vi "RRR_Joystick_Control_2025.vi"() -> ()   [LabVIEW 2020]
uses:
  <vilib>/MakerHub/LINX/Public/Peripherals/Analog/Analog Read N Chans.vi
  <vilib>/MakerHub/LINX/Public/Peripherals/Digital/Digital Read N Chans.vi
  <vilib>/MakerHub/LINX/Private/Local IO/LinxAnalogRead.vi
  <vilib>/MakerHub/LINX/Public/Utilities/Check Channel.vi
  <vilib>/MakerHub/LINX/Private/Local IO/LinxDigitalRead.vi
  <vilib>/MakerHub/LINX/Public/Utilities/Open Serial.vi
  <vilib>/MakerHub/LINX/Private/Utilties/Generate Error.vi
  <vilib>/MakerHub/LINX/LMH-LINX.lvlib
panel:
  out "Claw Angale":ext(slide) scale=0.0..1.0
  in  "Digital Channels":u8[](array[numeric])=[6, 7]
  in  "Analog Channels":u8[](array[numeric])=[0, 1, 2, 3]
  in  "Stop Button 2":bool
  out "Loop Rate (Hz) 2":u32=4294967295
  out "Voltages":dbl[](array[numeric])
  out "Values":bool[](array[boolean])
  out "Joint1_Theta":dbl=-2.0
  out "Joint2_Theta":dbl=-2.0
  out "Joint3_Theta":dbl=-2.0
  out "Claw_Theta":dbl=-2.0
  in  "Serial Port":refnum<visa-resource-name>="COM10"
  in  "Base position  Y":dbl
  in  "Base position X":dbl
  in  "Scale Factor":dbl(slide)=0.7 scale=0.5..1.0
  out "RRR - Forward Kinematics Visual":picture
  in  "Add details":bool=TRUE
  in  "Light Direction":dbl(knob)=5.611498737356196 scale format="%#.1f"
  in  "Colors":T1={"Joint 1"=16750848, "Arm 1"=16764006, "Joint 2"=26316, "Arm B"=6723993, "Joint 4"=16724787, "Claw"=16776960, "Joint 3"=26316, "Arm C"=6723993}
  out "TCP_Y":dbl=-5.928238312801877
  out "Joint2_Y":dbl=-3.8376690474488075
  out "Joint1_Y":dbl=-1.7449748351250485
  out "TCP_X":dbl=99.78690076611498
  out "Joint2_X":dbl=79.89646285874952
  out "Joint1_X":dbl=49.969541350954785
  in  "Arm 3":dbl=20.0
  out "RRR - Forward Kinematics":cluster{dbl[], dbl[]}(graph)={[0.0, 49.969541350954785, 79.89646285874952, 99.78690076611498], [39.0, -1.7449748351250485, -3.8376690474488075, -5.928238312801877]}
  in  "Arm 2":dbl=30.0
  in  "Arm 1":dbl=50.0
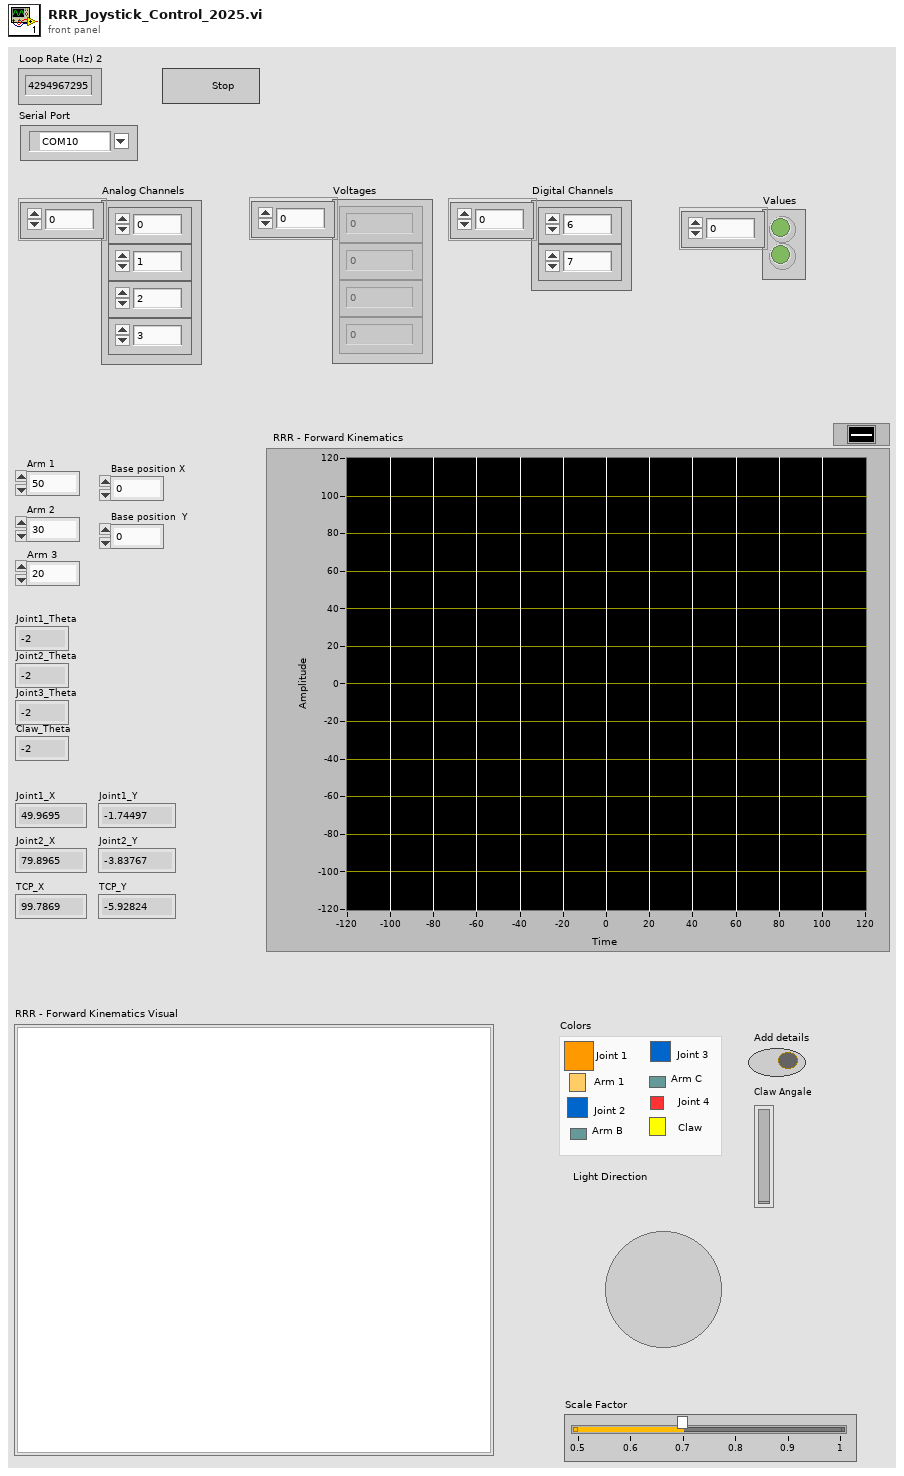
[diagram p1: front panel]
types:
  T1 = cluster{"Joint 1":u32, "Arm 1":u32, "Joint 2":u32, "Arm B":u32, "Joint 4":u32, "Claw":u32, "Joint 3":u32, "Arm C":u32}
  T2 = typedef "LMH-LINX.lvlib/LINX Ref.ctl" = cluster{"IO":T3, "Interface":T4, "LINX Device Config":T5}
  T3 = typedef "LMH-LINX.lvlib/Platform.ctl" = enum16{"Remote", "Local"}
  T4 = typedef "LMH-LINX.lvlib/Interface.ctl" = enum16{"Serial", "TCP"}
  T5 = typedef "LMH-LINX.lvlib/Device.lvlib/LINX Device Config.ctl" = cluster{"Interface":T4, "COM Port":refnum<visa-resource-name>, "TCP Configuration":T6, "Device Family":u8, "Device ID":u8, "Device Name":string, "TCP Ref":refnum<k5>, "Channels":T7}
  T6 = typedef "LMH-LINX.lvlib/Device.lvlib/TCP Config.ctl" = cluster{"IP Address":string, "Port":u16}
  T7 = typedef "LMH-LINX.lvlib/Channels.ctl" = cluster{"DI":u8[], "DO":u8[], "AI":u8[], "AO":u8[], "PWM":u8[], "QE":u8[], "UART":u8[], "I2C 2":u8[], "SPI":u8[], "CAN":u8[], "Servo":u8[], "AI Ref (V)":dbl, "AI Resolution (Bits)":u8, "AO Ref (V)":dbl, "AO Resolution (Bits)":u8}
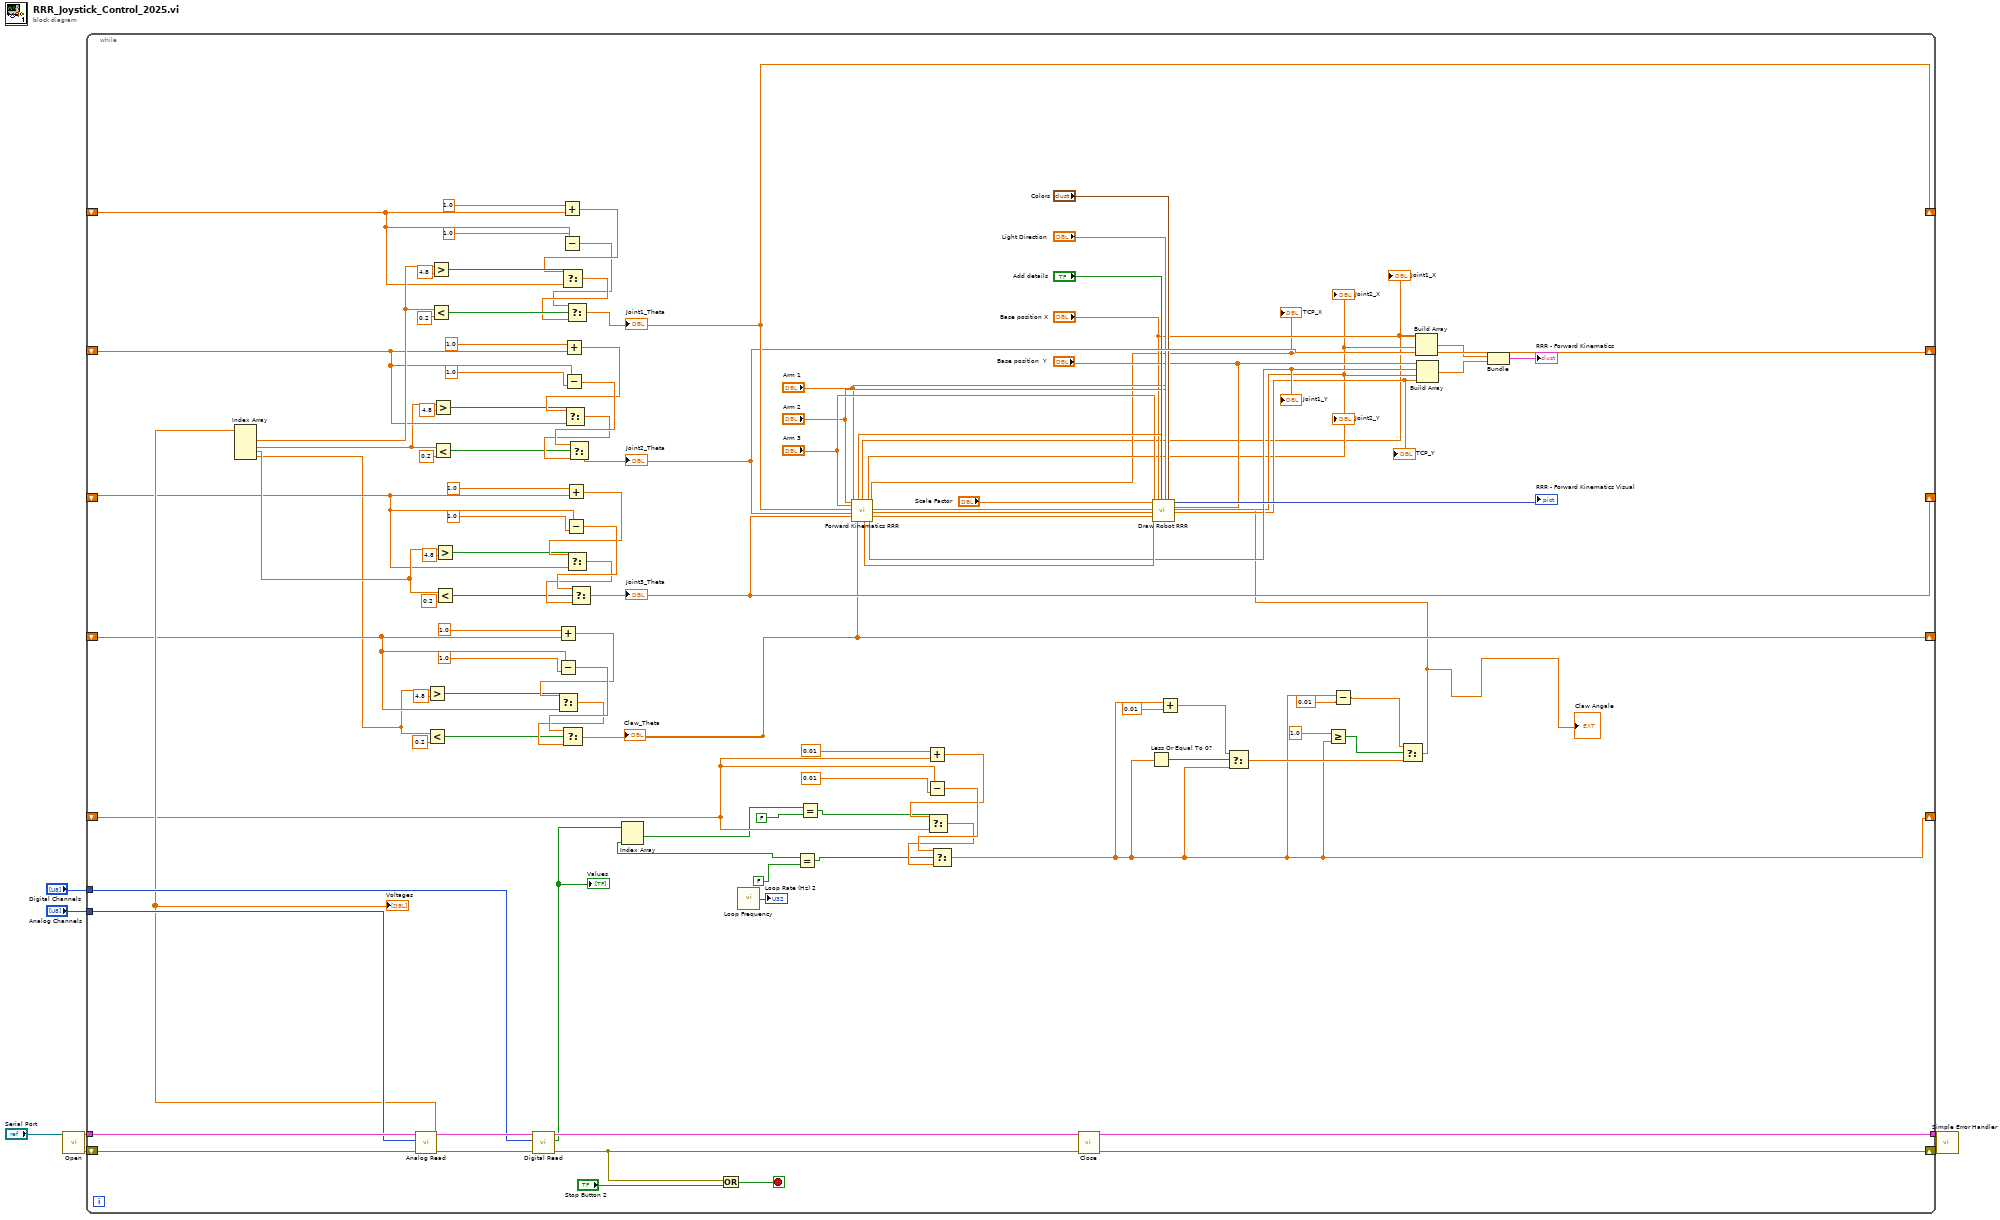
[diagram p0: block diagram]
diagram:
  n1 = call-poly <vilib>:"Open.vi"("Serial Port"="Serial Port") -> ("Error Out"=w7:errorcluster, "LINX Resource"=w8:T2)  [unwired: 8 in, 1 out]
  n2 = while {
    tunnel: w8 -> [w111]
    tunnel: [w108] -> w6
    shift-right: [w107] -> w5
    shift-left: w7 -> [w105]
    tunnel: "Analog Channels" -> [w110]
    tunnel: "Digital Channels" -> [w104]
    shift-right: [w58] -> _
    shift-left: _ -> [w92]
    shift-right: [w57] -> _
    shift-left: _ -> [w82]
    shift-right: [w56] -> _
    shift-left: _ -> [w70]
    shift-right: [w55] -> _
    shift-left: _ -> [w60]
    shift-right: [w10] -> _
    shift-left: _ -> [w25]
    stop <- w114 stop-if-true
    n3 = call-poly <vilib>:"Analog Read.vi"("Error In"=w105, "AI Channel(s)"=w110, "LINX Resource"=w111) -> ("Error Out"=w106:errorcluster, "Voltages"=w103:dbl[], "LINX Resource"=w109:T2)  [unwired: 5 in, 1 out]
    "Voltages" <- w103
    n4 = Index Array(array=w103) -> (element #1=w102:dbl, element #2=w81:dbl, element #3=w71:dbl, element #4=w59:dbl)  [unwired: 4 in]
    n5 = Greater?(x=w59, y=4.8) -> (0:w65:bool)
    n6 = Less?(x=w59, y=0.2) -> (x < y?=w66:bool)
    n7 = Greater?(x=w102, y=4.8) -> (0:w99:bool)
    n8 = Less?(x=w102, y=0.2) -> (x < y?=w98:bool)
    n9 = Greater?(x=w81, y=4.8) -> (0:w87:bool)
    n10 = Less?(x=w81, y=0.2) -> (x < y?=w88:bool)
    n11 = Greater?(x=w71, y=4.8) -> (0:w76:bool)
    n12 = Less?(x=w71, y=0.2) -> (x < y?=w77:bool)
    n13 = call-poly <vilib>:"Digital Read.vi"("Error In"=w106, "DI Channels"=w104, "LINX Resource"=w109) -> ("Error Out"=w107:errorcluster, "Values"=w31:bool[], "LINX Resource"=w108:T2)  [unwired: 6 in]
    "Values" <- w31
    n14 = Add(x=1.0 ("t"), y=w60) -> (x+y=w68:dbl)
    n15 = Subtract(x=w60, y=1.0 ("t")) -> (x-y=w69:dbl)
    n16 = Select(t=w68, s=w65, f=w60) -> (s? t:f=w67:dbl)
    n17 = Add(x=1.0 ("t"), y=w92) -> (x+y=w95:dbl)
    n18 = Subtract(x=w92, y=1.0 ("t")) -> (x-y=w94:dbl)
    n19 = Select(t=w95, s=w99, f=w92) -> (s? t:f=w97:dbl)
    n20 = Select(t=w69, s=w66, f=w67) -> (s? t:f=w55:dbl)
    "Claw_Theta" <- w55
    n21 = Add(x=1.0 ("t"), y=w82) -> (x+y=w90:dbl)
    n22 = Subtract(x=w82, y=1.0 ("t")) -> (x-y=w91:dbl)
    n23 = Select(t=w90, s=w87, f=w82) -> (s? t:f=w89:dbl)
    n24 = Add(x=1.0 ("t"), y=w70) -> (x+y=w79:dbl)
    n25 = Subtract(x=w70, y=1.0 ("t")) -> (x-y=w80:dbl)
    n26 = Select(t=w94, s=w98, f=w97) -> (s? t:f=w58:dbl)
    "Joint1_Theta" <- w58
    n27 = Select(t=w79, s=w76, f=w70) -> (s? t:f=w78:dbl)
    n28 = Select(t=w91, s=w88, f=w89) -> (s? t:f=w57:dbl)
    "Joint2_Theta" <- w57
    n29 = Select(t=w80, s=w77, f=w78) -> (s? t:f=w56:dbl)
    "Joint3_Theta" <- w56
    n30 = Index Array(array=w31) -> (element #1=w21:bool, element #2=w22:bool)  [unwired: 2 in]
    n31 = Or(x=w107, y="Stop Button 2") -> (x .or. y?=w114:bool)
    n32 = call <vilib>:"Loop Frequency.vi"() -> ("Loop Rate (Hz)"=→"Loop Rate (Hz) 2":u32)
    n33 = Equal?(x=w22, y=FALSE) -> (x = y?=w23:bool)
    n34 = Equal?(x=w21, y=FALSE) -> (x = y?=w24:bool)
    n35 = call "Forward Kinematics RRR.vi"("Arm in"="Arm 2", "Arm 3"="Arm 3", "Joint 1"=w58, "Joint in"=w57, "Joint 3"=w56, "Arm 1"="Arm 1", "Claw Angle"=w55) -> ("Numeric"=w49:dbl, "x1"=w32:dbl, "Numeric 2"=w47:dbl, "x2"=w37:dbl, "Numeric 3"=w44:dbl, "x_final"=w36:dbl, "y1"=w40:dbl, "y2"=w38:dbl, "y_final"=w39:dbl, "Numeric 4"=w41:dbl)  [unwired: 3 in]
    "Joint1_X" <- w32
    "Joint2_X" <- w37
    "TCP_X" <- w36
    "Joint1_Y" <- w40
    "Joint2_Y" <- w38
    "TCP_Y" <- w39
    n36 = Add(x=0.01 ("t"), y=w25) -> (x+y=w29:dbl)
    n37 = Subtract(x=w25, y=0.01 ("t")) -> (x-y=w30:dbl)
    n38 = Select(t=w29, s=w24, f=w25) -> (s? t:f=w28:dbl)
    n39 = Select(t=w30, s=w23, f=w28) -> (s? t:f=w10:dbl)
    n40 = Less Or Equal To 0?(x=w10) -> (x <= 0?=w18:bool)
    n41 = Add(x=w10, y=0.01 ("t")) -> (x+y=w16:dbl)
    n42 = Select(t=w16, s=w18, f=w10) -> (s? t:f=w11:dbl)
    n43 = Greater Or Equal?(x=1.0, y=w10) -> (x >= y?=w12:bool)
    n44 = Subtract(x=w10, y=0.01 ("t")) -> (x-y=w15:dbl)
    n45 = Select(t=w15, s=w12, f=w11) -> (s? t:f=w9:dbl)
    "Claw Angale" <- w9
    n46 = call "Draw Robot RRR.vi"("Scale Factor"="Scale Factor", "Base position  Y"="Base position  Y", "Claw Value"=w9, "Numeric 4"=w41, "Arm 3"="Arm 3", "Numeric 3"=w44, "Base position X"="Base position X", "Numeric 2"=w47, "Add details"="Add details", "Numeric"=w49, "Light Direction"="Light Direction", "Arm 1"="Arm 1", "Colors"="Colors", "Arm in"="Arm 2") -> ("Picture Out"=→"RRR - Forward Kinematics Visual":picture)  [unwired: 5 in]
    n47 = Build Array("Base position X", w32, w37, w36) -> (w33:dbl[])
    n48 = Build Array("Base position  Y", w40, w38, w39) -> (w34:dbl[])
    n49 = Bundle(w33, w34) -> (→"RRR - Forward Kinematics":cluster{dbl[], dbl[]})  [unwired: 1 in]
  }
  n50 = call <vilib>:"Close.vi"("Error In"=w5, "LINX Resource"=w6) -> ("Error Out"=w3:errorcluster)  [unwired: 9 in]
  n51 = call <vilib>:"Simple Error Handler.vi"("error in (no error)"=w3) -> ()  [unwired: 4 in, 5 out]
